vi "UE9 PWM16 and Duty Cycle.vi"(8 "error in":errorcluster, 9 "PWM Duty Cycle [%]":dbl=50.0 format="%.4f") -> (0 "error out":errorcluster)   [LabVIEW 2021]
panel:
  in  "Case Constant\n(See Context Help)":bool=TRUE
  out "Measured Duty Cycle [%]":dbl format="%.8f"
  out "Low Time (s)":dbl format="%.8f"
  out "Low Time (Clocks)":u16
  out "High Time (s)":dbl format="%.8f"
  out "High Time (Clocks)":u16
  out "Timer1 Value Read":u32
  in  "FirstFound":bool=TRUE
  in  "Address":string="1"
  out "Error Message":string
  # "Demonstrates 1 timer channel of 16-bit PWM output with a frequency of 40.6 Hz, and 1 timer channel doing\nduty cycle input.  Short FIO0 (PWM output) to FIO1 (duty cycle input) and then you can measure the duty\ncycle of the output."
  # "USB"
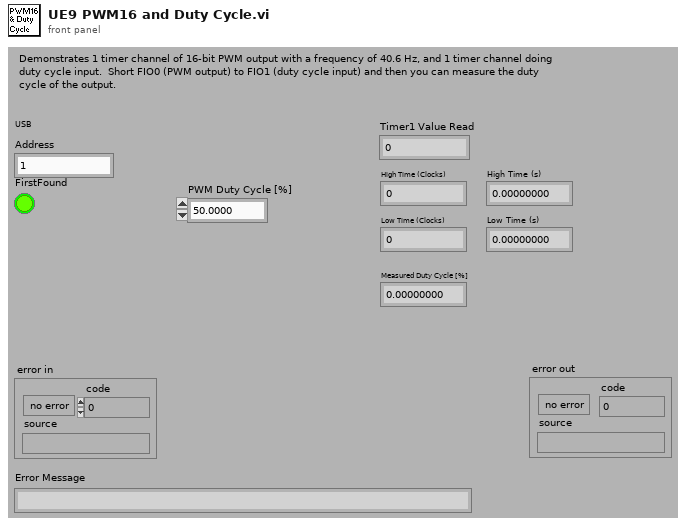
[diagram p1: front panel]
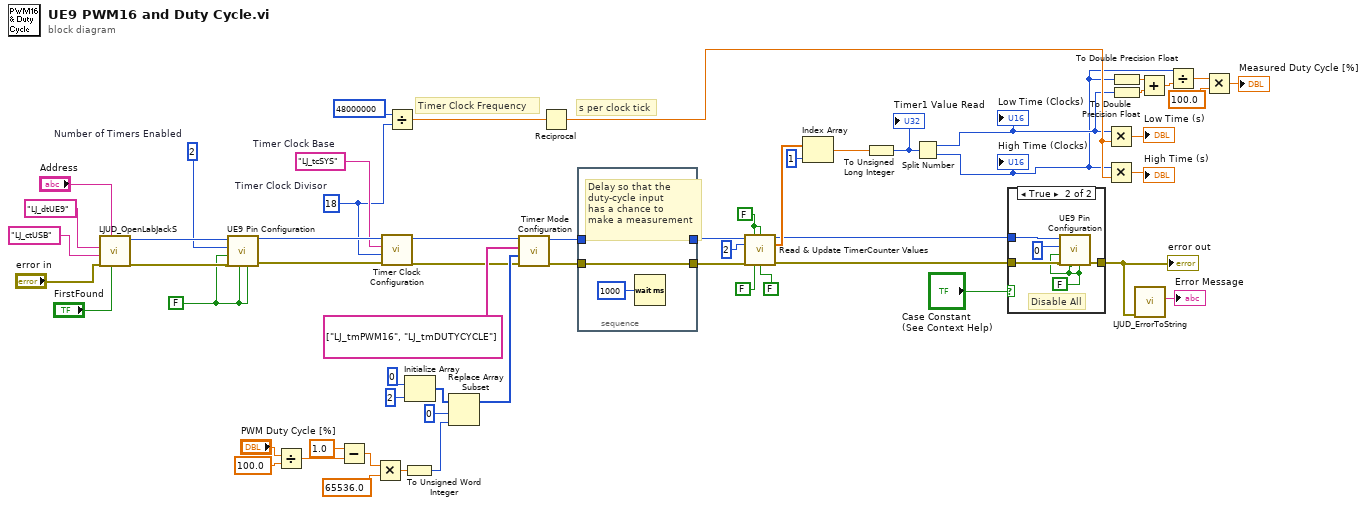
[diagram p0: block diagram]
diagram:
  w17 = 18  # Timer Clock Divisor
  w19 = "LJ_tcSYS"  # Timer Clock Base
  w29 = u8 2  # Number of Timers Enabled
  w27 = FALSE ("Enable Counter0")
  w49 = FALSE ("Reset Counter0")
  # "s per clock tick"
  # "Timer Clock Frequency"
  n1 = call "LJUD_OpenLabJackS.vi"("FirstFound"="FirstFound", "Address"="Address", "error in"="error in", "ConnectionType"="LJ_ctUSB", "DeviceType"="LJ_dtUE9") -> ("error out"=w37:errorcluster, "Handle"=w38:i32)  [unwired: 4 in, 1 out]
  n2 = call "UE9 Pin Configuration.vi"("Enable Counter1"=w27, "Enable Counter0"=w27, "error in"=w37, "Enable DACs"=w27, "Number of Timers Enabled"=w29, "Handle In"=w38) -> ("error out"=w34:errorcluster, "Handle Out"=w33:i32)  [unwired: 4 in]
  n3 = Divide(x="PWM Duty Cycle [%]", y=100.0) -> (x/y=w54:dbl)
  n4 = Subtract(x=1.0, y=w54) -> (x-y=w52:dbl)
  n5 = Multiply(x=w52, y=65536.0) -> (x*y=w26:dbl)
  n6 = call "Timer Clock Configuration.vi"("error in"=w34, "Timer Clock Divisor"=w17, "Timer Clock Base"=w19, "Handle In"=w33) -> ("error out"=w35:errorcluster, "Handle Out"=w32:i32)  [unwired: 6 in]
  n7 = Divide(x=48000000, y=w17) -> (x/y=w15:dbl)
  n8 = To Unsigned Word Integer(number=w26) -> (unsigned 16bit integer=w25:u16)
  n9 = Initialize Array(u16 0 ("PWM Timer Value"), 2 ("Dimension Size")) -> (w42:u16[])
  n10 = Replace Array Subset(array=w42, new element=w25, index=0 ("Index")) -> (w36:u16[])
  n11 = call "Timer Mode Configuration.vi"("error in"=w35, "TimerValues"=w36, "TimerModes"=string[] ["LJ_tmPWM16", "LJ_tmDUTYCYCLE"], "Handle In"=w32) -> ("error out"=w24:errorcluster, "Handle Out"=w22:i32)  [unwired: 6 in]
  n12 = Reciprocal(x=w15) -> (1/x=w14:dbl)
  n13 = stacked-sequence {
    tunnel: w24 -> [w62]
    tunnel: [w62] -> w23
    tunnel: w22 -> [w61]
    tunnel: [w61] -> w21
    frame #0 {
      # "Delay so that the\nduty-cycle input\nhas a chance to\nmake a measurement"
      n14 = Wait (ms)(milliseconds to wait=u32 1000) -> ()  [unwired: 1 out]
    }
  }
  n15 = call "Read & Update TimerCounter Values.vi"("Handle In"=w21, "Reset Counter0"=w49, "Reset Counter1"=w49, "# Timers to Read"=2, "error in"=w23, "Read Counter0"=FALSE ("Reset Counter0"), "Read Counter1"=FALSE ("Reset Counter0")) -> ("Handle Out"=w3:i32, "Timer Value Reads"=w20:dbl[], "error out"=w2:errorcluster)  [unwired: 5 in, 1 out]
  n16 = Index Array(array=w20, index=1 ("Index")) -> (element=w1:dbl)
  n17 = To Unsigned Long Integer(number=w1) -> (unsigned 32bit integer=w16:u32)
  "Timer1 Value Read" <- w16
  n18 = Split Number(x=w16) -> (hi(x)=w8:u16, lo(x)=w7:u16)
  "High Time (Clocks)" <- w7
  "Low Time (Clocks)" <- w8
  n19 = case shown="True" "Case Constant\n(See Context Help)" {
    tunnel: w2 -> [w63 w68]
    tunnel: w3 -> [_ w67]
    tunnel: [w63 w66] -> w46
    frame False {
    }
    frame True {
      w64 = FALSE ("Enable Counter0")
      # "Disable All"
      n20 = call "UE9 Pin Configuration.vi"("Enable Counter1"=w64, "Enable Counter0"=w64, "error in"=w68, "Enable DACs"=w64, "Number of Timers Enabled"=0 ("# Timers Enabled"), "Handle In"=w67) -> ("error out"=w66:errorcluster)  [unwired: 4 in, 1 out]
    }
  }
  "error out" <- w46
  n21 = Multiply(x=w8, y=w14) -> (x*y=→"Low Time (s)":dbl)
  n22 = Multiply(x=w7, y=w14) -> (x*y=→"High Time (s)":dbl)
  n23 = To Double Precision Float(number=w7) -> (double precision float=w9:dbl)
  n24 = To Double Precision Float(number=w8) -> (double precision float=w10:dbl)
  n25 = call "LJUD_ErrorToString.vi"("error in"=w46) -> ("String"=→"Error Message":string)  [unwired: 10 in]
  n26 = Add(x=w9, y=w10) -> (x+y=w11:dbl)
  n27 = Divide(x=w7, y=w11) -> (x/y=w6:dbl)
  n28 = Multiply(x=w6, y=100.0) -> (x*y=→"Measured Duty Cycle [%]":dbl)
